vi "DSF.Engine.Transceiver Thread.New.vi"(8 "error in (no error)":errorcluster, 10 "Cache":refnum<class "DSF.Engine.Memory.Cache.lvclass">, 11 "Transceiver type":refnum<class "DSF.Engine.Transceiver.lvclass">) -> (0 "error out":errorcluster, 3 "Transceiver Thread out":refnum<class "DSF.Engine.Transceiver Thread.lvclass">)   [LabVIEW 2017, in "DSF.Engine.lvlib" / "DSF.Engine.Transceiver Thread.lvclass"]
uses:
  DSF.Engine.Transceiver Thread.lvclass
  DSF.Engine.Transceiver.lvclass
  Cache/DSF.Engine.Memory.Cache.lvclass
  DSF.Engine.Transceiver Thread.lvclass/DSF.Engine.Transceiver Thread.ctl
  Interface/DSF.Engine.Interface.Transceiver.lvclass
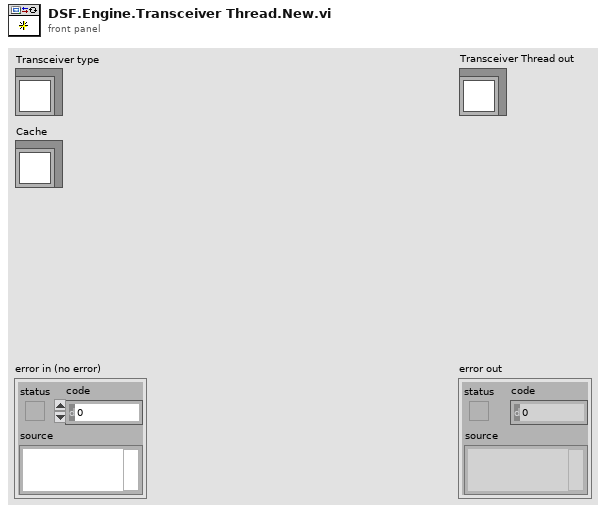
[diagram p1: front panel]
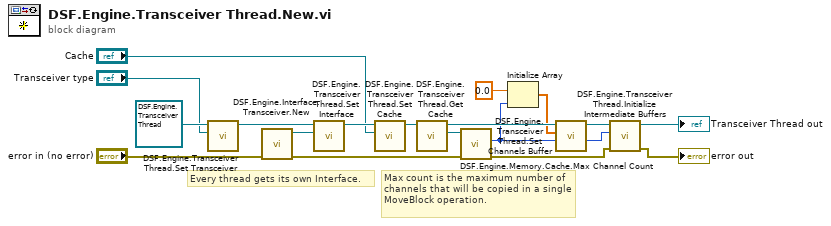
[diagram p0: block diagram]
diagram:
  # "Max count is the maximum number of channels that will be copied in a single MoveBlock operation."
  # "Every thread gets its own Interface."
  n1 = call "DSF.Engine.Transceiver Thread.Set Transceiver.vi"("Transceiver"="Transceiver type", "Transceiver Thread in"=refnum<class "DSF.Engine.Transceiver Thread.lvclass"> refnum) -> ("Transceiver Thread out"=w14:refnum<class "DSF.Engine.Transceiver Thread.lvclass">)  [unwired: 9 in]
  n2 = call "DSF.Engine.Interface.Transceiver.New.vi"("error in (no error)"="error in (no error)") -> ("error out"=w9:errorcluster, "Transceiver Interface"=w15:refnum<class "DSF.Engine.Interface.Transceiver.lvclass">)  [unwired: 9 in]
  n3 = call "DSF.Engine.Transceiver Thread.Set Interface.vi"("Interface"=w15, "Transceiver Thread in"=w14) -> ("Transceiver Thread out"=w13:refnum<class "DSF.Engine.Transceiver Thread.lvclass">)  [unwired: 9 in]
  n4 = call "DSF.Engine.Transceiver Thread.Set Cache.vi"("Cache"="Cache", "Transceiver Thread in"=w13) -> ("Transceiver Thread out"=w11:refnum<class "DSF.Engine.Transceiver Thread.lvclass">)  [unwired: 9 in]
  n5 = call "DSF.Engine.Transceiver Thread.Get Cache.vi"("Transceiver Thread in"=w11) -> ("Cache"=w10:refnum<class "DSF.Engine.Memory.Cache.lvclass">, "Transceiver Thread out"=w7:refnum<class "DSF.Engine.Transceiver Thread.lvclass">)  [unwired: 9 in]
  n6 = call "DSF.Engine.Memory.Cache.Max Channel Count.vi"("error in (no error)"=w9, "Cache in"=w10) -> ("error out"=w2:errorcluster, "max channel count"=w4:u64)  [unwired: 7 in, 1 out]
  n7 = Initialize Array(0.0 ("element"), w4) -> (w6:dbl[])
  n8 = call "DSF.Engine.Transceiver Thread.Set Channels Buffer.vi"("channels buffer"=w6, "Transceiver Thread in"=w7) -> ("Transceiver Thread out"=w5:refnum<class "DSF.Engine.Transceiver Thread.lvclass">)  [unwired: 9 in]
  n9 = call "DSF.Engine.Transceiver Thread.Initialize Intermediate Buffers.vi"("error in (no error)"=w2, "channel count"=w4, "Transceiver Thread in"=w5) -> ("error out"=→"error out":errorcluster, "Transceiver Thread out"=→"Transceiver Thread out":refnum<class "DSF.Engine.Transceiver Thread.lvclass">)  [unwired: 7 in]
